vi "Highlight Trace.vi"(8 "error in (no error)":errorcluster, 10 "Trace":i32, 11 "Graph Manager in":refnum<class "Graph Manager.lvclass">) -> (0 "error out":errorcluster, 3 "Graph Manager out":refnum<class "Graph Manager.lvclass">)   [LabVIEW 2016, in "Graph Manager.lvclass"]
uses:
  Graph Manager.lvclass
  Graph Manager.lvclass/Graph Manager.ctl
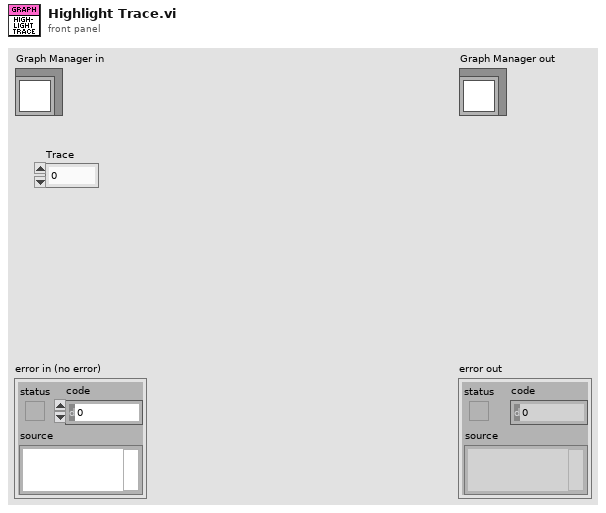
[diagram p1: front panel]
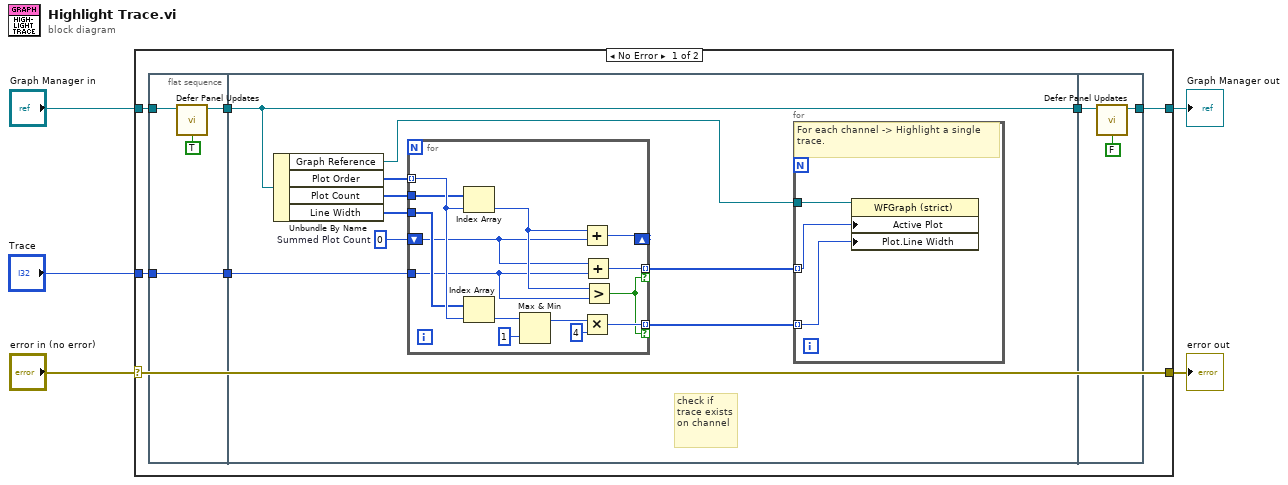
[diagram p0: block diagram]
diagram:
  n1 = case shown="No Error" "error in (no error)" {
    selector: "error in (no error)" -> [w12 w47]
    tunnel: [w12 w47] -> w4
    tunnel: [w9 w46] -> w2
    tunnel: "Graph Manager in" -> [w11 w46]
    tunnel: "Trace" -> [w10 _]
    frame No Error {
      n2 = flat-sequence {
        tunnel: w10 -> [w16]
        tunnel: w11 -> [w15]
        tunnel: [w14] -> w7
        tunnel: [w16] -> w6
        tunnel: [w17] -> w8
        tunnel: w7 -> [w17]
        tunnel: w6 -> [w21]
        tunnel: [w44] -> w9
        tunnel: w8 -> [w45]
        frame #0 {
          n3 = call-dynamic "Defer Panel Updates.vi"("Defer Panel Updates"=TRUE, "Graph Manager in"=w15) -> ("Graph Manager out"=w14:refnum<class "Graph Manager.lvclass">)  [unwired: 8 in, 1 out]
        }
        frame #1 {
          w20 = 0  # Summed Plot Count
          # "check if trace exists on channel"
          n4 = Unbundle By Name(w17) -> ("Graph Reference"=w25:refnum<vi>, "Plot Order"=w24:i32[], "Plot Count"=w23:i32[], "Line Width"=w22:u8[])
          n5 = for {
            tunnel: w24 -> [w38] mode=indexing
            tunnel: w23 -> [w37]
            tunnel: w22 -> [w36]
            tunnel: [w34] -> w18 mode=indexing if=w29
            tunnel: w21 -> [w30]
            shift-right: [w33] -> _
            shift-left: w20 -> [w32]
            tunnel: [w31] -> w19 mode=indexing if=w29
            n6 = Index Array(array=w37, index=w38) -> (element=w39:i32)
            n7 = Index Array(array=w36, index=w38) -> (element=w28:u8)
            n8 = Max & Min(x=w28, y=u8 1) -> (max(x,y)=w26:u8)  [unwired: 1 out]
            n9 = Add(x=w39, y=w32) -> (x+y=w33:i32)
            n10 = Multiply(x=w26, y=u8 4) -> (x*y=w34:u8)
            n11 = Add(x=w32, y=w30) -> (x+y=w31:i32)
            n12 = Greater?(x=w39, y=w30) -> (0:w29:bool)
          }
          n13 = for {
            tunnel: w25 -> [w42]
            tunnel: w19 -> [w41] mode=indexing
            tunnel: w18 -> [w40] mode=indexing
            # "For each channel -> Highlight a single trace."
            n14 = property class="WFGraph (strict)"(reference=w42, "Active Plot"=w41, "Plot.Line Width"=w40) -> ()  [unwired: 1 in, 2 out]
          }
        }
        frame #2 {
          n15 = call-dynamic "Defer Panel Updates.vi"("Defer Panel Updates"=FALSE, "Graph Manager in"=w45) -> ("Graph Manager out"=w44:refnum<class "Graph Manager.lvclass">)  [unwired: 8 in, 1 out]
        }
      }
    }
    frame Error {
    }
  }
  "error out" <- w4
  "Graph Manager out" <- w2
